vi "Handle Last Ack Core.vi"(4 "error in (no error)":errorcluster, 6 "Last Ack":refnum<class "Last Ack.lvclass">, 7 "CS++StartActor in":refnum<class "CS++StartActor.lvclass">) -> (0 "error out":errorcluster, 3 "CS++StartActor out":refnum<class "CS++StartActor.lvclass">)   [LabVIEW 2015, in "CS++StartActor.lvlib" / "CS++StartActor.lvclass"]
doc: "(<B>Filename</B>: Actor Framework.lvlib:Actor.lvclass:Handle Last Ack Core.vi)\n\nDefines how the caller actor responds to the Last Ack message from a nested actor. The Last Ack message is the final message a nested actor sends to its caller before it shuts down. The message contains information about the final state of the nested actor.\n\nBy default, this method does nothing except return any error the nested actor sent. A descendant class may override this method to define behavior."
uses:
  CS++StartActor.lvclass
  <vilib>/ActorFramework/LastAck/Last Ack.lvclass
  <vilib>/ActorFramework/Actor/Actor.lvclass/Actor.ctl
  <vilib>/ActorFramework/Message Enqueuer/Message Enqueuer.lvclass/Message Enqueuer.ctl
  CS++StartActor.lvclass/CS++StartActor.ctl
  <vilib>/ActorFramework/Message Enqueuer/Init from Existing Queue.vi
  <vilib>/ActorFramework/Message Enqueuer/Enqueue.vi
  <vilib>/ActorFramework/Message Priority Queue/Priority Enqueue.vi
  <vilib>/ActorFramework/Stop Msg/Stop Msg.lvclass
  <vilib>/ActorFramework/Message Enqueuer/Message Enqueuer.lvclass
  <vilib>/ActorFramework/Actor/Actor.lvclass
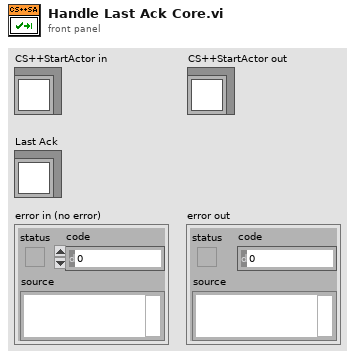
[diagram p1: front panel]
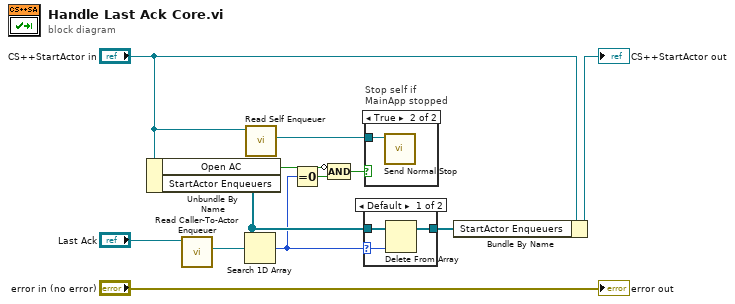
[diagram p0: block diagram]
diagram:
  n1 = Unbundle By Name("CS++StartActor in") -> ("Open AC"=w9:bool, "StartActor Enqueuers"=w5:refnum<class "Message Enqueuer.lvclass">[])
  n2 = call <vilib>:"Read Caller-To-Actor Enqueuer.vi"("Last Ack"="Last Ack") -> ("Caller-to-Actor Enqueuer"=w11:refnum<class "Message Enqueuer.lvclass">)  [unwired: 10 in]
  n3 = Search 1D Array(1D array=w5, element=w11) -> (index of element=w4:i32)  [unwired: 1 in]
  n4 = call <vilib>:"Read Self Enqueuer.vi"("Actor"="CS++StartActor in") -> ("Self Enqueuer"=w10:refnum<class "Message Enqueuer.lvclass">)  [unwired: 10 in]
  n5 = Equal To 0?(x=w4) -> (x = 0?=w8:bool)
  n6 = Compound Arithmetic op=AND(invert w9, w8) -> (w7:bool)
  n7 = case shown="Default" w4 {
    selector: w4 -> [w14 _]
    tunnel: w5 -> [w15 w16]
    tunnel: [w13 w16] -> w3
    frame Default {
      n8 = Delete From Array(array=w15, index=w14) -> (array with subset deleted=w13:refnum<class "Message Enqueuer.lvclass">[])  [unwired: 1 in, 1 out]
    }
    frame -1 {
    }
  }
  n9 = case "Stop self if\nMainApp stopped" shown="True" w7 {
    tunnel: w10 -> [_ w17]
    frame False {
    }
    frame True {
      n10 = call <vilib>:"Send Normal Stop.vi"("Message Enqueuer"=w17) -> ()  [unwired: 10 in, 1 out]
    }
  }
  n11 = Bundle By Name(cluster="CS++StartActor in", "StartActor Enqueuers"=w3) -> (→"CS++StartActor out":refnum<class "CS++StartActor.lvclass">)
  "error out" <- "error in (no error)"
